vi "Kiwi_Set_Refnum.vi"(8 "error in (no error)":errorcluster, 10 "refnum name":string, 11 "Kiwi DevRef In":T1={"Motor A"={"DeviceStatus"={"status"=FALSE, "code"=0, "source"=""}, "Type"=enum."PWM", "PWM"={"PWM Channel"=enum."Invalid", "DeadBand"={"Name"="", "maxPositivePwm"=0, "minPositivePwm"=0, "centerPwm"=0, "maxNegativePwm"=0, "minNegativePwm"=0, "angularRange"=0}}, "CAN"={"Device Number"=0, "Control Mode"=enum."Percent VBus", "Semaphore"=refnum, "Max Vout"=12.0, "TalonSRX Control Mode"=enum."Percent VBus"}, "Invert"=FALSE}, "Motor B"={"DeviceStatus"={"status"=FALSE, "code"=0, "source"=""}, "Type"=enum."PWM", "PWM"={"PWM Channel"=enum."Invalid", "DeadBand"={"Name"="", "maxPositivePwm"=0, "minPositivePwm"=0, "centerPwm"=0, "maxNegativePwm"=0, "minNegativePwm"=0, "angularRange"=0}}, "CAN"={"Device Number"=0, "Control Mode"=enum."Percent VBus", "Semaphore"=refnum, "Max Vout"=12.0, "TalonSRX Control Mode"=enum."Percent VBus"}, "Invert"=FALSE}, "Motor C"={"DeviceStatus"={"status"=FALSE, "code"=0, "source"=""}, "Type"=enum."PWM", "PWM"={"PWM Channel"=enum."Invalid", "DeadBand"={"Name"="", "maxPositivePwm"=0, "minPositivePwm"=0, "centerPwm"=0, "maxNegativePwm"=0, "minNegativePwm"=0, "angularRange"=0}}, "CAN"={"Device Number"=0, "Control Mode"=enum."Percent VBus", "Semaphore"=refnum, "Max Vout"=12.0, "TalonSRX Control Mode"=enum."Percent VBus"}, "Invert"=FALSE}, "Config Consts"={"Arx"=0.0, "Ay"=0.0, "Brx"=0.0, "By"=0.0, "Cr"=0.0, "Cy"=0.0, "Cx"=0.0, "MaxMotorVal"=0.0}, "status"={"status"=FALSE, "code"=0, "source"=""}, "Angles"={"Angle A"=60.0, "Angle B"=60.0, "Angle C"=60.0, "Radians?"=FALSE}, "MotorVals"={"MotorA"=0.0, "MotorB"=0.0, "MotorC"=0.0}}) -> (0 "error out":errorcluster, 3 "Kiwi DevRef Out":T1={"Motor A"={"DeviceStatus"={"status"=FALSE, "code"=0, "source"=""}, "Type"=enum."PWM", "PWM"={"PWM Channel"=enum."Invalid", "DeadBand"={"Name"="", "maxPositivePwm"=0, "minPositivePwm"=0, "centerPwm"=0, "maxNegativePwm"=0, "minNegativePwm"=0, "angularRange"=0}}, "CAN"={"Device Number"=0, "Control Mode"=enum."Percent VBus", "Semaphore"=refnum, "Max Vout"=12.0, "TalonSRX Control Mode"=enum."Percent VBus"}, "Invert"=FALSE}, "Motor B"={"DeviceStatus"={"status"=FALSE, "code"=0, "source"=""}, "Type"=enum."PWM", "PWM"={"PWM Channel"=enum."Invalid", "DeadBand"={"Name"="", "maxPositivePwm"=0, "minPositivePwm"=0, "centerPwm"=0, "maxNegativePwm"=0, "minNegativePwm"=0, "angularRange"=0}}, "CAN"={"Device Number"=0, "Control Mode"=enum."Percent VBus", "Semaphore"=refnum, "Max Vout"=12.0, "TalonSRX Control Mode"=enum."Percent VBus"}, "Invert"=FALSE}, "Motor C"={"DeviceStatus"={"status"=FALSE, "code"=0, "source"=""}, "Type"=enum."PWM", "PWM"={"PWM Channel"=enum."Invalid", "DeadBand"={"Name"="", "maxPositivePwm"=0, "minPositivePwm"=0, "centerPwm"=0, "maxNegativePwm"=0, "minNegativePwm"=0, "angularRange"=0}}, "CAN"={"Device Number"=0, "Control Mode"=enum."Percent VBus", "Semaphore"=refnum, "Max Vout"=12.0, "TalonSRX Control Mode"=enum."Percent VBus"}, "Invert"=FALSE}, "Config Consts"={"Arx"=0.0, "Ay"=0.0, "Brx"=0.0, "By"=0.0, "Cr"=0.0, "Cy"=0.0, "Cx"=0.0, "MaxMotorVal"=0.0}, "status"={"status"=FALSE, "code"=0, "source"=""}, "Angles"={"Angle A"=60.0, "Angle B"=60.0, "Angle C"=60.0, "Radians?"=FALSE}, "MotorVals"={"MotorA"=0.0, "MotorB"=0.0, "MotorC"=0.0}})   [LabVIEW 2015]
uses:
  <userlib>/836-Library/Drive/kiwi/support/Kiwi_Dev_Ref.ctl
  <vilib>/Rock Robotics/WPI/MotorControl/WPI_MotorControlDeviceRef.ctl
  <vilib>/Rock Robotics/WPI/MotorControl/WPI_MotorControlType.ctl
  <vilib>/Rock Robotics/SystemInterfaces/DIO/FPGA_DIOPWMChannel.ctl
  <vilib>/Rock Robotics/WPI/PWM/WPI_PWMDeadband.ctl
  <vilib>/Rock Robotics/WPI/CAN/Jaguar/SubVIs/WPI_CANJaguar_ControlMode.ctl
  <vilib>/Rock Robotics/WPI/CAN/TalonSRX/WPI_CANTalonSRX_APIControlMode.ctl
  <userlib>/836-Library/Drive/kiwi/support/Kiwi_Cal_Constants.ctl
  <userlib>/836-Library/Drive/kiwi/support/Kiwi_Angles.ctl
  <vilib>/Rock Robotics/WPI/Utilities/Refnum Registry Operation.ctl
panel:
  out "refnum names":string[](array[string])
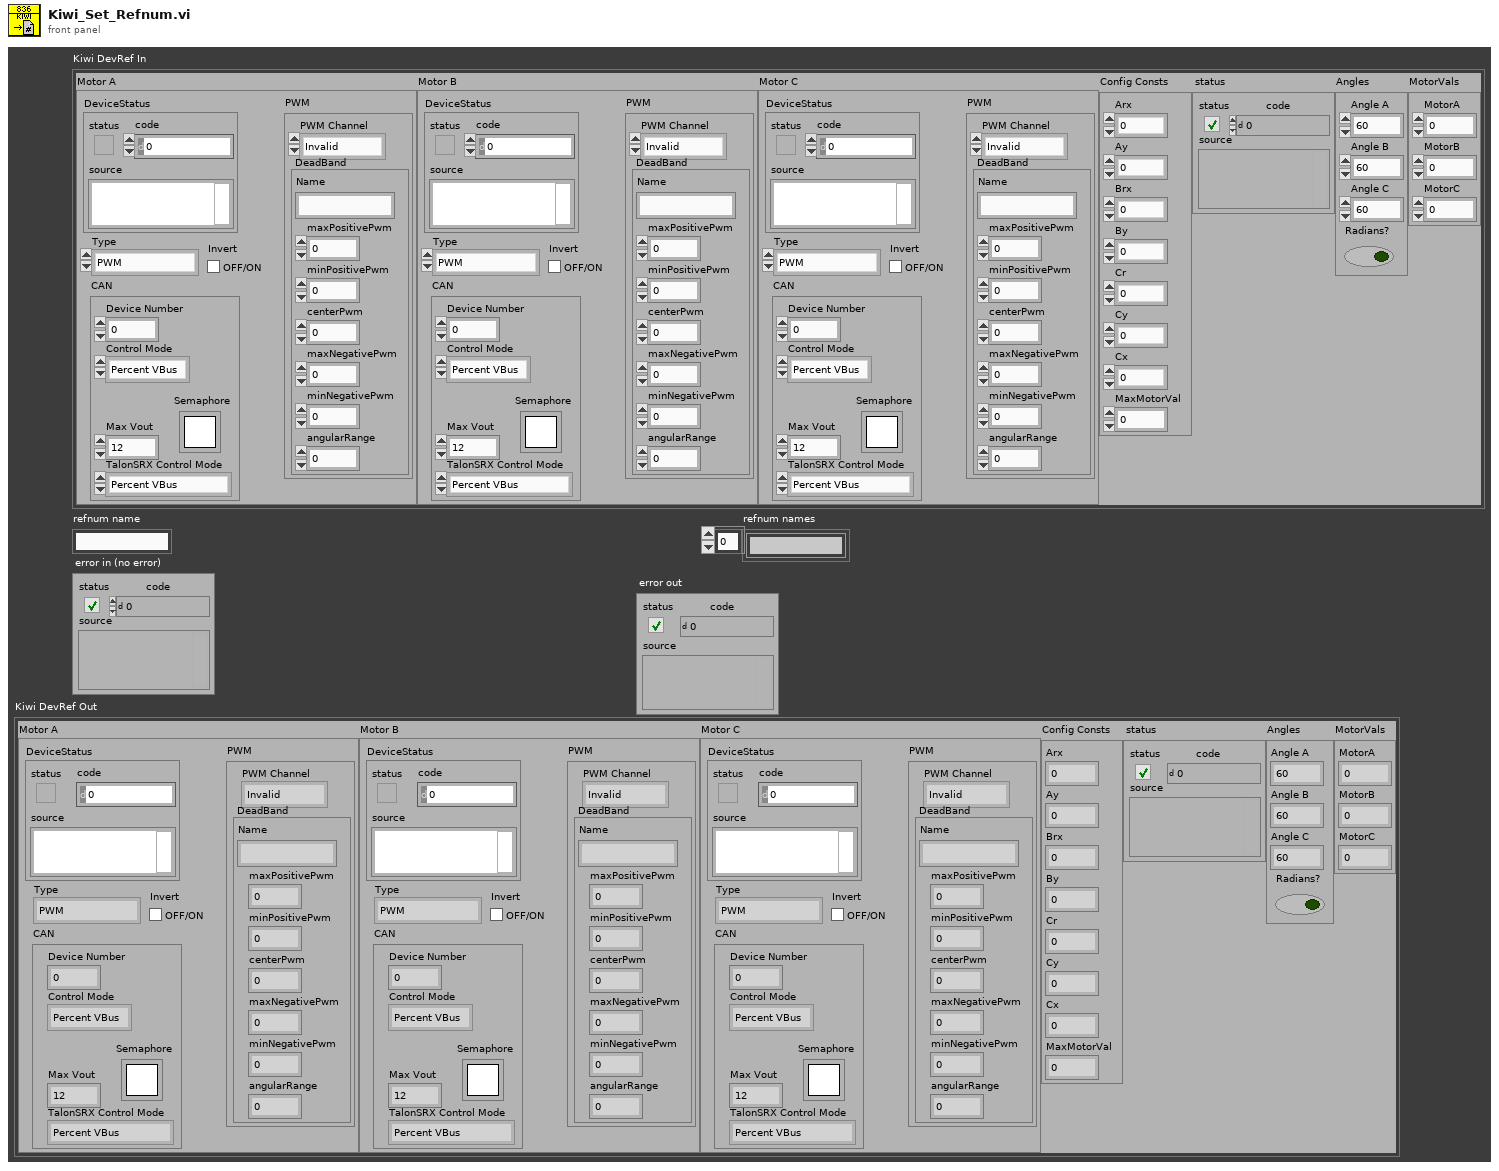
[diagram p1: front panel]
types:
  T1 = typedef "Kiwi_Dev_Ref.ctl" = cluster{"Motor A":T2, "Motor B":T2, "Motor C":T2, "Config Consts":T9, "status":errorcluster, "Angles":T10, "MotorVals":cluster{"MotorA":dbl, "MotorB":dbl, "MotorC":dbl}}
  T2 = typedef "WPI_MotorControlDeviceRef.ctl" = cluster{"DeviceStatus":errorcluster, "Type":T3, "PWM":cluster{"PWM Channel":T4, "DeadBand":T5}, "CAN":cluster{"Device Number":u8, "Control Mode":T6, "Semaphore":T7, "Max Vout":dbl, "TalonSRX Control Mode":T8}, "Invert":bool}
  T3 = typedef "WPI_MotorControlType.ctl" = enum16{"PWM", "CAN", "CANTalonSRX"}
  T4 = typedef "FPGA_DIOPWMChannel.ctl" = enum8{"PWM 0", "PWM 1", "PWM 2", "PWM 3", "PWM 4", "PWM 5", "PWM 6", "PWM 7", "PWM 8", "PWM 9", "PWM MXP 0", "PWM MXP 1", "PWM MXP 2", "PWM MXP 3", "PWM MXP 4", "PWM MXP 5", "PWM MXP 6", "PWM MXP 7", "PWM MXP 8", "PWM MXP 9", "Invalid"}
  T5 = typedef "WPI_PWMDeadband.ctl" = cluster{"Name":string, "maxPositivePwm":i32, "minPositivePwm":i32, "centerPwm":i32, "maxNegativePwm":i32, "minNegativePwm":i32, "angularRange":u16}
  T6 = typedef "WPI_CANJaguar_ControlMode.ctl" = enum8{"Percent VBus", "Current", "Speed", "Position", "Voltage"}
  T7 = typedef "Semaphore RefNum" = refnum<k1>
  T8 = typedef "WPI_CANTalonSRX_APIControlMode.ctl" = enum8{"Percent VBus", "Speed", "Position", "Slave", "Unchanged / Invalid", "Voltage Compensation", "Current", "Motion Profile"}
  T9 = typedef "Kiwi_Cal_Constants.ctl" = cluster{"Arx":dbl, "Ay":dbl, "Brx":dbl, "By":dbl, "Cr":dbl, "Cy":dbl, "Cx":dbl, "MaxMotorVal":dbl}
  T10 = typedef "Kiwi_Angles.ctl" = cluster{"Angle A":dbl, "Angle B":dbl, "Angle C":dbl, "Radians?":bool}
  T11 = typedef "Refnum Registry Operation.ctl" = enum16{"set", "get", "delete", "get all names", "read name"}
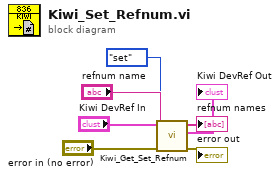
[diagram p0: block diagram]
diagram:
  n1 = call <userlib>:"Kiwi_Get_Set_Refnum.vi"("error in (no error)"="error in (no error)", "menu"=Refnum_Registry_Operation."set", "refnum name"="refnum name", "Kiwi DevRef In"="Kiwi DevRef In") -> ("error out"=→"error out":errorcluster, "Kiwi DevRef Out"=→"Kiwi DevRef Out":T1, "refnum names"=→"refnum names":string[])  [unwired: 5 in]
